vi "2sincos.vi"() -> ()   [LabVIEW 2013]
uses:
  <vilib>/rvi/FXPMathLib/FxpSinAndCos/subVIs/nifxpmath_SinAndCos_SimConfig.ctl
  <vilib>/rvi/FXPMathLib/FxpSinAndCos/simVIs/DllFxpSinAndCosTemp_sub.vi
  <vilib>/rvi/FXPMathLib/FxpSinAndCos/XNode/nifxpmath_SinAndCos.xnode
panel:
  in  "input valid":bool=TRUE
  in  "x in":fxp<+/-,32,4>
  out "output valid":bool
  out "cos_fi_korr":fxp<+/-,16,2>
  out "sin fi_korr":fxp<+/-,16,2>
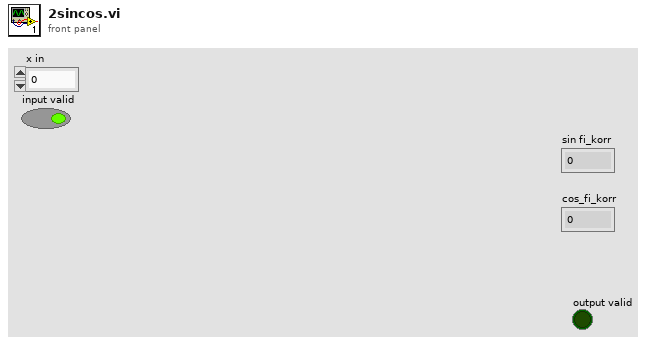
[diagram p1: front panel]
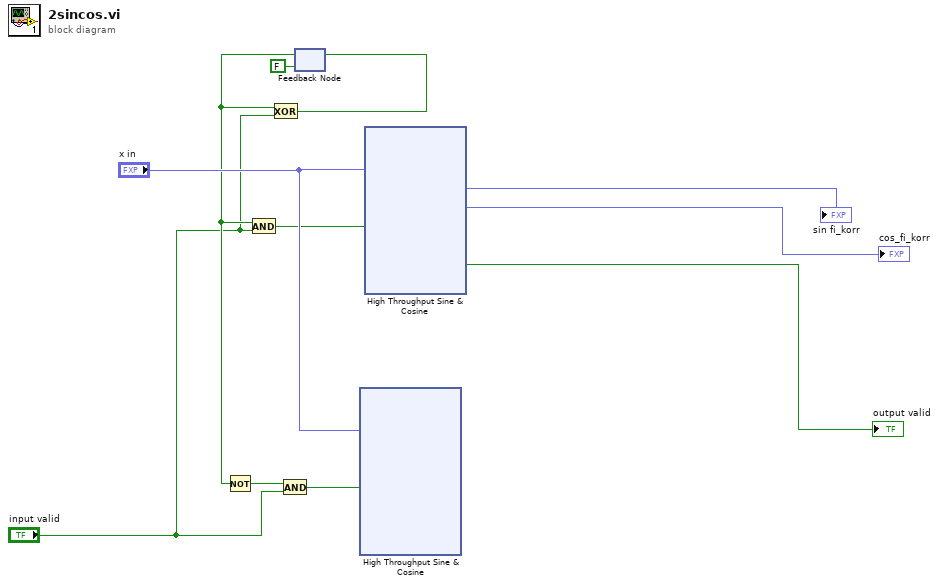
[diagram p0: block diagram]
diagram:
  n1 = feedback #1(FALSE) -> (w4:bool)
  n2 = Not(x=w4) -> (.not. x?=w3:bool)
  n3 = And(x=w4, y="input valid") -> (x .and. y?=w7:bool)
  n4 = Exclusive Or(1:"input valid", 2:w4) -> (0:w6:bool)
  n5 = And(x=w3, y="input valid") -> (x .and. y?=w1:bool)
  n6 = feedback-in #1(w6) -> ()
  n7 = xnode "High Throughput Sine & Cosine"("x (pi)"="x in", "input valid"=w1) -> ()  [unwired: 1 in, 4 out]
  n8 = xnode "High Throughput Sine & Cosine"("x (pi)"="x in", "input valid"=w7) -> ("sin(x)"=→"sin fi_korr":fxp<+/-,16,2>, "cos(x)"=→"cos_fi_korr":fxp<+/-,16,2>, "output valid"=→"output valid":bool)  [unwired: 1 in, 1 out]
